vi "Init File Load Dialog Data.vi"(8 "error in (no error)":errorcluster, 11 "Node Ptr":T1 format="%.0x") -> (0 "error out":errorcluster, 3 "FileDialog":T2={"File"=path "", "Group"="", "Channel"="", "DataPlugin"="", "MissingTeeth"=0.0, "ErrState"="", "File Selected"=FALSE, "Data Selection Method"=enum."Manual", "Offset"=0, "Length"=0, "DataPlugins Info"=[], "Controls"=[], "File Ref"=refnum, "Groups"=[], "Channels"=[], "Groups Refs"=[], "Channel Refs"=[], "Cancelled"=FALSE, "Position reference"=enum."Crank angle", "FPGA memory size"=enum."32,768", "GroupRef"=refnum, "ChanRef"=refnum, "Data"=[], "ReverseData"=FALSE, "DispTwoRotations"=FALSE, "cycle range"=720})   [LabVIEW 2019, in "Engine Simulation Toolkit System Explorer.lvlib"]
uses:
  Engine Simulation Toolkit System Explorer.lvlib
  File Load Dialog.ctl
  Data Replay Data Selection Method.ctl
  <vilib>/Platform/storage/utility/usiPluginInformation.ctl
  Position Reference.ctl
  FPGA Mem Size.ctl
  <vilib>/NI VeriStand/Custom Device API/Custom Device Item Ref.ctl
  Shared/Properties.vi
  <vilib>/NI VeriStand/Custom Device API/Get Item Property (Dependent File).vi
  <vilib>/NI VeriStand/Custom Device API/Get Item Property (U16).vi
  <vilib>/NI VeriStand/Custom Device API/Get Item Property (String).vi
  <vilib>/NI VeriStand/Custom Device API/Get Item Property (Double).vi
  <vilib>/NI VeriStand/Custom Device API/Get Item Property (U32).vi
  <vilib>/NI VeriStand/Custom Device API/Get Item Property (Boolean).vi
  <vilib>/NI VeriStand/Custom Device API/Custom Device API.lvlib
  Shared/Engine Simulation Toolkit Shared.lvlib
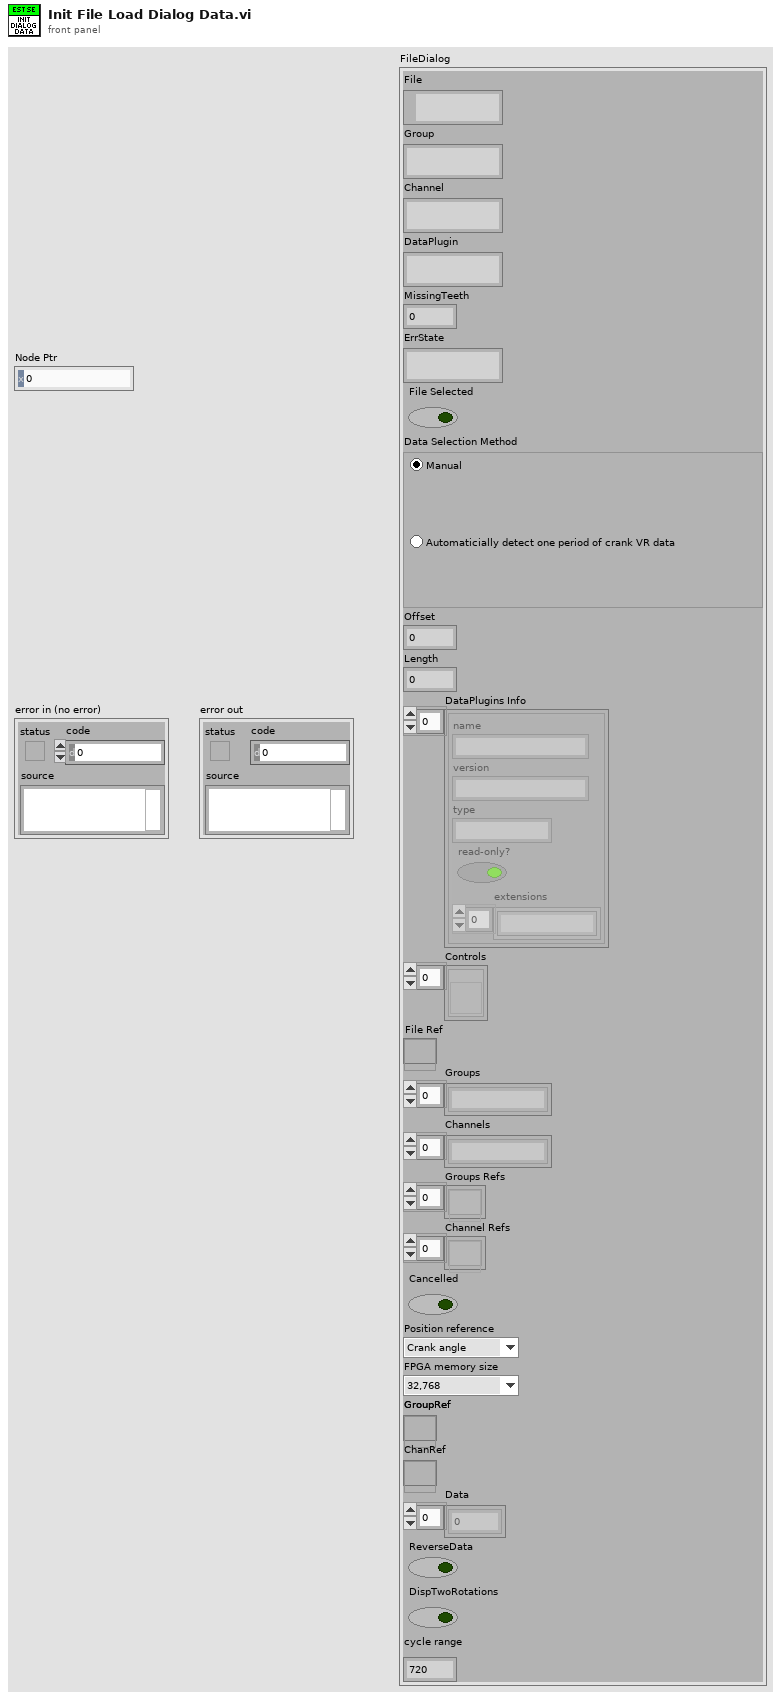
[diagram p1: front panel]
types:
  T1 = typedef "Custom Device API.lvlib/Custom Device Item Ref.ctl" = u64
  T2 = typedef "Engine Simulation Toolkit System Explorer.lvlib/File Load Dialog.ctl" = cluster{"File":path, "Group":string, "Channel":string, "DataPlugin":string, "MissingTeeth":dbl, "ErrState":string, "File Selected":bool, "Data Selection Method":T3, "Offset":i32, "Length":i32, "DataPlugins Info":T4[], "Controls":refnum<vi>[], "File Ref":refnum<k20>, "Groups":string[], "Channels":string[], "Groups Refs":refnum<k20>[], "Channel Refs":refnum<k20>[], "Cancelled":bool, "Position reference":T5, "FPGA memory size":T6, "GroupRef":refnum<k20>, "ChanRef":refnum<k20>, "Data":dbl[], "ReverseData":bool, "DispTwoRotations":bool, "cycle range":u16}
  T3 = typedef "Engine Simulation Toolkit System Explorer.lvlib/Data Replay Data Selection Method.ctl" = enum32{"Manual", "AutoVRCrank"}
  T4 = typedef "usiPluginInformation.ctl" = cluster{"name":string, "version":string, "type":string, "read-only?":bool, "extensions":string[]}
  T5 = typedef "Engine Simulation Toolkit System Explorer.lvlib/Position Reference.ctl" = enum16{"Crank angle", "Cycle angle"}
  T6 = typedef "Engine Simulation Toolkit System Explorer.lvlib/FPGA Mem Size.ctl" = enum16{"65,536", "32,768", "16,384", "8,192", "4,096", "2,048", "1,024"}
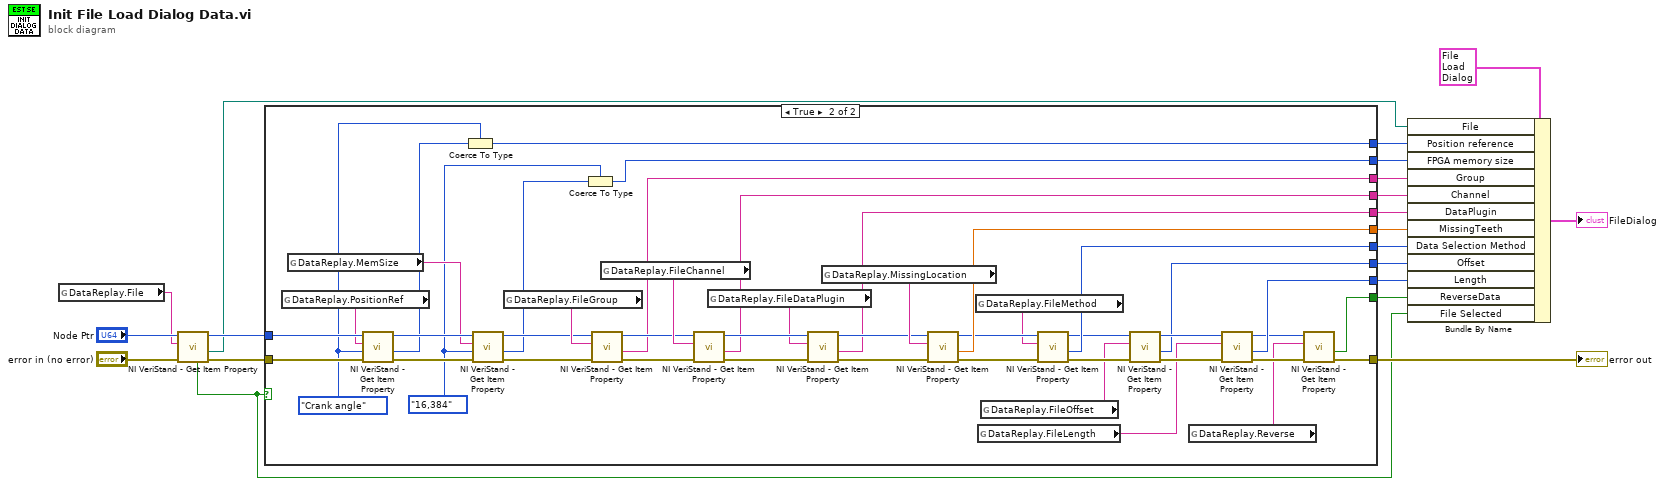
[diagram p0: block diagram]
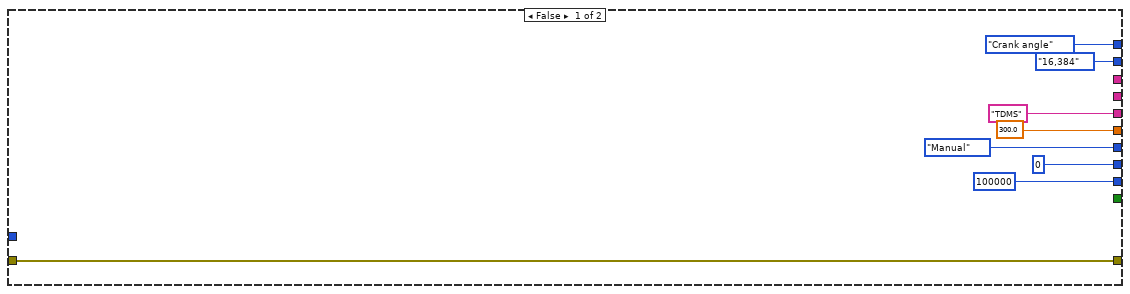
[diagram p2: hidden frame]
diagram:
  n1 = global read "Properties.vi" "DataReplay.File"() -> (w5:string)
  n2 = call-poly <vilib>:"NI VeriStand - Get Item Property.vi"("error in (no error)"="error in (no error)", "Property Name"=w5, "Item Ref in"="Node Ptr") -> ("error out"=w13:errorcluster, "Path"=w7:path, "Item Ref out"=w12:T1, "Found"=w3:bool)  [unwired: 4 in, 1 out]
  n3 = case shown="True" w3 {
    tunnel: w12 -> [_ w38]
    tunnel: w13 -> [w26 w73]
    tunnel: [w26 w45] -> w20
    tunnel: [_ w62] -> w15
    tunnel: [_ w61] -> w16
    tunnel: ["TDMS" ("Default Value") w60] -> w17
    tunnel: [300.0 w59] -> w18
    tunnel: [Data_Replay_Data_Selection_Method."Manual" ("Data Selection Method") w55] -> w10
    tunnel: [u32 0 ("Value") w47] -> w9
    tunnel: [u32 100000 ("Value") w46] -> w8
    tunnel: [_ w42] -> w4
    tunnel: [Position_Reference."Crank angle" ("Position reference") w30] -> w2
    tunnel: [FPGA_Mem_Size."16,384" ("FPGA memory size") w32] -> w1
    frame False {
    }
    frame True {
      w29 = Position_Reference."Crank angle" ("Position reference")
      w33 = FPGA_Mem_Size."16,384" ("FPGA memory size")
      n4 = global read "Properties.vi" "DataReplay.PositionRef"() -> (w36:string)
      n5 = global read "Properties.vi" "DataReplay.MemSize"() -> (w35:string)
      n6 = call-poly <vilib>:"NI VeriStand - Get Item Property.vi"("error in (no error)"=w73, "Default Value"=w29, "Property Name"=w36, "Item Ref in"=w38) -> ("error out"=w39:errorcluster, "Value"=w31:u16, "Item Ref out"=w37:T1)  [unwired: 4 in, 1 out]
      n7 = Coerce To Type(0:w31, 1:w29) -> (2:w30:T5)
      n8 = call-poly <vilib>:"NI VeriStand - Get Item Property.vi"("error in (no error)"=w39, "Default Value"=w33, "Property Name"=w35, "Item Ref in"=w37) -> ("error out"=w41:errorcluster, "Value"=w34:u16, "Item Ref out"=w40:T1)  [unwired: 4 in, 1 out]
      n9 = global read "Properties.vi" "DataReplay.FileGroup"() -> (w72:string)
      n10 = Coerce To Type(0:w34, 1:w33) -> (2:w32:T6)
      n11 = call-poly <vilib>:"NI VeriStand - Get Item Property.vi"("error in (no error)"=w41, "Property Name"=w72, "Item Ref in"=w40) -> ("error out"=w69:errorcluster, "Value"=w62:string, "Item Ref out"=w70:T1)  [unwired: 5 in, 1 out]
      n12 = global read "Properties.vi" "DataReplay.FileChannel"() -> (w71:string)
      n13 = call-poly <vilib>:"NI VeriStand - Get Item Property.vi"("error in (no error)"=w69, "Property Name"=w71, "Item Ref in"=w70) -> ("error out"=w67:errorcluster, "Value"=w61:string, "Item Ref out"=w68:T1)  [unwired: 5 in, 1 out]
      n14 = global read "Properties.vi" "DataReplay.FileDataPlugin"() -> (w66:string)
      n15 = call-poly <vilib>:"NI VeriStand - Get Item Property.vi"("error in (no error)"=w67, "Property Name"=w66, "Item Ref in"=w68) -> ("error out"=w63:errorcluster, "Value"=w60:string, "Item Ref out"=w64:T1)  [unwired: 5 in, 1 out]
      n16 = global read "Properties.vi" "DataReplay.MissingLocation"() -> (w65:string)
      n17 = call-poly <vilib>:"NI VeriStand - Get Item Property.vi"("error in (no error)"=w63, "Property Name"=w65, "Item Ref in"=w64) -> ("error out"=w57:errorcluster, "Value"=w59:dbl, "Item Ref out"=w58:T1)  [unwired: 5 in, 1 out]
      n18 = global read "Properties.vi" "DataReplay.FileMethod"() -> (w56:string)
      n19 = global read "Properties.vi" "DataReplay.FileLength"() -> (w48:string)
      n20 = global read "Properties.vi" "DataReplay.FileOffset"() -> (w49:string)
      n21 = call-poly <vilib>:"NI VeriStand - Get Item Property.vi"("error in (no error)"=w57, "Property Name"=w56, "Item Ref in"=w58) -> ("error out"=w53:errorcluster, "Value"=w55:u32, "Item Ref out"=w54:T1)  [unwired: 5 in, 1 out]
      n22 = call-poly <vilib>:"NI VeriStand - Get Item Property.vi"("error in (no error)"=w53, "Property Name"=w49, "Item Ref in"=w54) -> ("error out"=w51:errorcluster, "Value"=w47:u32, "Item Ref out"=w52:T1)  [unwired: 5 in, 1 out]
      n23 = global read "Properties.vi" "DataReplay.Reverse"() -> (w43:string)
      n24 = call-poly <vilib>:"NI VeriStand - Get Item Property.vi"("error in (no error)"=w51, "Property Name"=w48, "Item Ref in"=w52) -> ("error out"=w50:errorcluster, "Value"=w46:u32, "Item Ref out"=w44:T1)  [unwired: 5 in, 1 out]
      n25 = call-poly <vilib>:"NI VeriStand - Get Item Property.vi"("error in (no error)"=w50, "Property Name"=w43, "Item Ref in"=w44) -> ("error out"=w45:errorcluster, "Value"=w42:bool)  [unwired: 5 in, 2 out]
    }
  }
  "error out" <- w20
  n26 = Bundle By Name(cluster=T2 {"File"=path "", "Group"="", "Channel"="", "DataPlugin"="", "MissingTeeth"=0.0, "ErrState"="", "File Selected"=FALSE, "Data Selection Method"=enum."Manual", "Offset"=0, "Length"=0, "DataPlugins Info"=[], "Controls"=[], "File Ref"=refnum, "Groups"=[], "Channels"=[], "Groups Refs"=[], "Channel Refs"=[], "Cancelled"=FALSE, "Position reference"=enum."Crank angle", "FPGA memory size"=enum."32,768", "GroupRef"=refnum, "ChanRef"=refnum, "Data"=[], "ReverseData"=FALSE, "DispTwoRotations"=FALSE, "cycle range"=0} ("FileDialog"), "File"=w7, "Position reference"=w2, "FPGA memory size"=w1, "Group"=w15, "Channel"=w16, "DataPlugin"=w17, "MissingTeeth"=w18, "Data Selection Method"=w10, "Offset"=w9, "Length"=w8, "ReverseData"=w4, "File Selected"=w3) -> (→"FileDialog":T2)
